vi "TSM SSC Digital Get HRAM Configuration.vi"(0 "Digital TSM In":T1, 11 "error in":errorcluster) -> (4 "Digital TSM Out":T1, 8 "HRAM Configuration":T3={"Finite Samples"=FALSE, "Cycles to Acquire"=2303, "Max Samples To Acquire Per Site"=8191, "Buffer Size Per Site"=32000, "Pretrigger Samples"=0, "Trigger Settings"={"Trigger Type"=2200, "Cycle Number Trigger:Cycle Number"=0, "Pattern Label Trigger:Pattern Label"="", "Pattern Label Trigger:Vector Offset"=0, "Pattern Label Trigger:Cycle Offset"=0}} {"Trigger Settings"."Trigger Type" items=["First Failure"=2200, "Cycle Number"=2201, "Pattern Label"=2202]; "Cycles to Acquire" items=["Failed Cycles"=2303, "All Cycles"=2304]}, 15 "error out":errorcluster)   [LabVIEW 2020]
uses:
  TSM/TSM SSC Digital.ctl
  <vilib>/NI_TestStand_SemiconductorModule/NI_TestStand_Semiconductor_Module.lvlibp/PinMap/Digital Pattern/PinQueryContext/DigitalPatternPinQueryContext.lvclass
  SSC Digital/SSC Digital.ctl
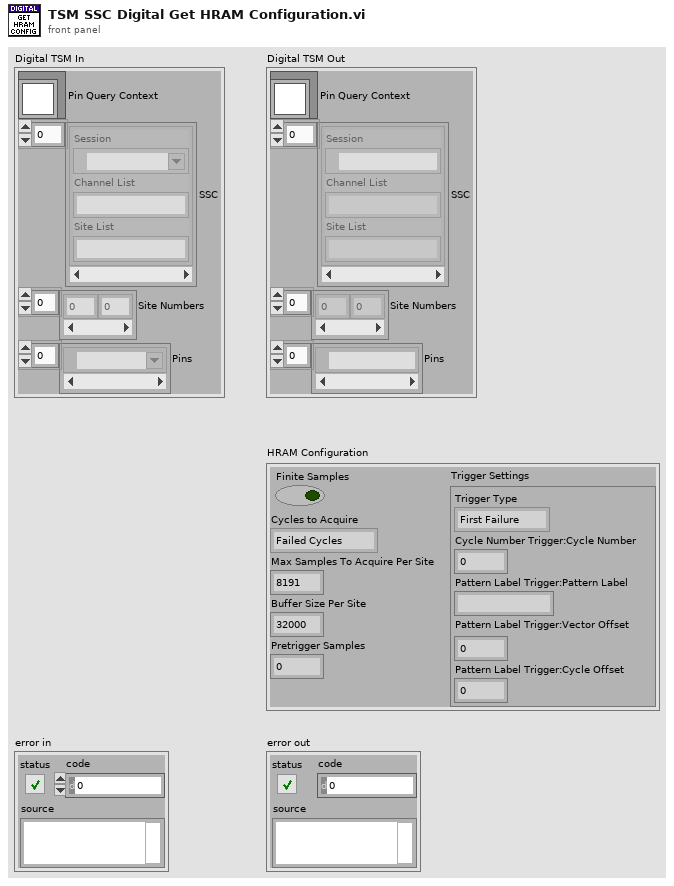
[diagram p1: front panel]
types:
  T1 = typedef "TSM SSC Digital.ctl" = cluster{"Pin Query Context":refnum<class "DigitalPatternPinQueryContext.lvclass">, "SSC":T2[], "Site Numbers":i32[], "Pins":tag[]}
  T2 = typedef "SSC Digital.ctl" = cluster{"Session":refnum<k15>, "Channel List":string, "Site List":string}
  T3 = cluster{"Finite Samples":bool, "Cycles to Acquire":i32, "Max Samples To Acquire Per Site":i32, "Buffer Size Per Site":i64, "Pretrigger Samples":i32, "Trigger Settings":cluster{"Trigger Type":i32, "Cycle Number Trigger:Cycle Number":i64, "Pattern Label Trigger:Pattern Label":string, "Pattern Label Trigger:Vector Offset":i64, "Pattern Label Trigger:Cycle Offset":i64}}
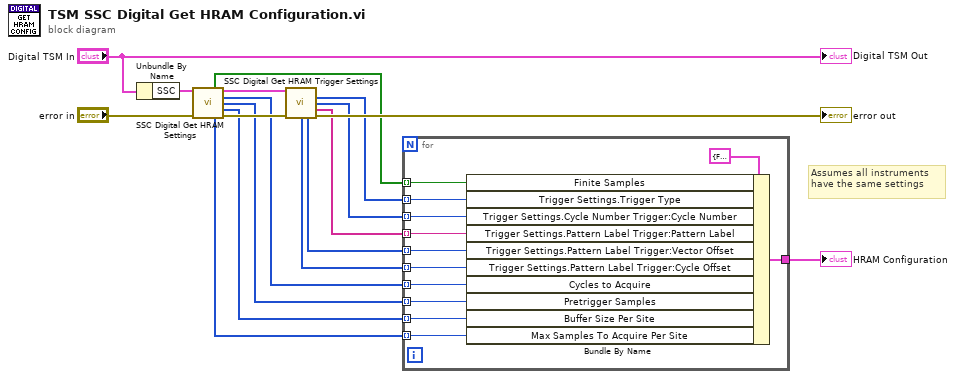
[diagram p0: block diagram]
diagram:
  # "Assumes all instruments have the same settings"
  n1 = Unbundle By Name("Digital TSM In") -> ("SSC"=w16:T2[])
  n2 = call "SSC Digital Get HRAM Settings.vi"("Digital SSC in"=w16, "error in"="error in") -> ("Per-Instrument Number of Samples is Finite"=w10:bool[], "Digital SSC out"=w12:T2[], "Per-Instrument Cycles to Acquire"=w9:i32[], "Per-Instrument Pretrigger Samples"=w8:i32[], "Per-Instrument Buffer Size Per Site"=w7:i64[], "Per-Instrument Max Samples To Acquire Per Site"=w6:i32[], "error out"=w14:errorcluster)  [unwired: 7 in]
  n3 = call "SSC Digital Get HRAM Trigger Settings.vi"("Digital SSC in"=w12, "error in"=w14) -> ("Per-Instrument Triggers Type"=w5:i32[], "Per-Instrument Cycle Number Trig:Cycle Number"=w4:i64[], "Per-Instrument Pattern Label Trig:Pattern Label"=w3:string[], "Per-Instrument Pattern Label Trig:Cycle Offset"=w1:i64[], "Per-Instrument Pattern Label Trig:Vector Offset"=w2:i64[], "error out"=→"error out":errorcluster)  [unwired: 7 in, 1 out]
  n4 = for {
    tunnel: w10 -> [w18] mode=indexing
    tunnel: w9 -> [w28] mode=indexing
    tunnel: w8 -> [w27] mode=indexing
    tunnel: w7 -> [w26] mode=indexing
    tunnel: w6 -> [w25] mode=indexing
    tunnel: w5 -> [w20] mode=indexing
    tunnel: w4 -> [w21] mode=indexing
    tunnel: w3 -> [w22] mode=indexing
    tunnel: w2 -> [w23] mode=indexing
    tunnel: w1 -> [w24] mode=indexing
    tunnel: [w29] -> w11
    n5 = Bundle By Name(cluster=T3 {"Finite Samples"=FALSE, "Cycles to Acquire"=2303, "Max Samples To Acquire Per Site"=0, "Buffer Size Per Site"=32000, "Pretrigger Samples"=0, "Trigger Settings"={"Trigger Type"=2200, "Cycle Number Trigger:Cycle Number"=0, "Pattern Label Trigger:Pattern Label"="", "Pattern Label Trigger:Vector Offset"=0, "Pattern Label Trigger:Cycle Offset"=0}} ("HRAM Configuration"), "Finite Samples"=w18, "Trigger Settings.Trigger Type"=w20, "Trigger Settings.Cycle Number Trigger:Cycle Number"=w21, "Trigger Settings.Pattern Label Trigger:Pattern Label"=w22, "Trigger Settings.Pattern Label Trigger:Vector Offset"=w23, "Trigger Settings.Pattern Label Trigger:Cycle Offset"=w24, "Cycles to Acquire"=w28, "Pretrigger Samples"=w27, "Buffer Size Per Site"=w26, "Max Samples To Acquire Per Site"=w25) -> (w29:T3)
  }
  "HRAM Configuration" <- w11
  "Digital TSM Out" <- "Digital TSM In"
